vi "CSMKVMapDVR.vi"(8 "error in (no error)":errorcluster) -> (0 "error out":errorcluster, 3 "KVMapDVR":refnum<data-value>)   [LabVIEW 2017, in "Communicable State Machine.lvlib"]
uses:
  Communicable State Machine.lvlib
  ChangeFlag/ChangeFlag-Write.vi
  Utility/Random Change Flag.vi
  ChangeFlag/ChangeFlagDB.vi
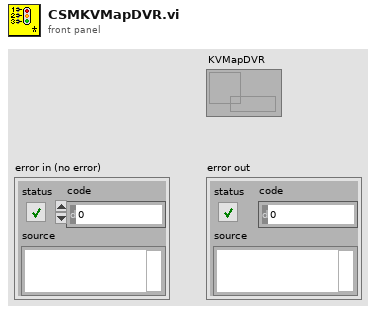
[diagram p1: front panel]
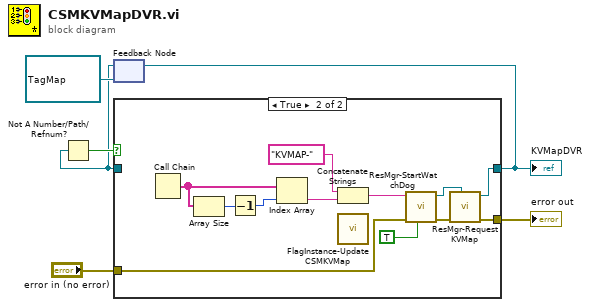
[diagram p0: block diagram]
diagram:
  n1 = feedback #1(refnum<data-value> refnum ("KVMapDVR")) -> (w3:refnum<data-value>)
  n2 = Not A Number/Path/Refnum?(number/path/refnum=w3) -> (NaN/Path/Refnum?=w4:bool)
  n3 = case shown="True" w4 {
    tunnel: w3 -> [w8 _]
    tunnel: [w8 w18] -> w6
    tunnel: [w7 w10] -> w2
    tunnel: "error in (no error)" -> [w7 w9]
    frame False {
    }
    frame True {
      n4 = Call Chain() -> (call chain=w13:string[])
      n5 = Array Size(array=w13) -> (size(s)=w12:i32)
      n6 = Decrement(x=w12) -> (x-1=w11:i32)
      n7 = Index Array(array=w13, index=w11) -> (element=w14:string)
      n8 = Concatenate Strings("KVMAP-" ("ModuleName"), w14) -> (w15:string)
      n9 = call "FlagInstance-Update CSMKVMap.vi"() -> ()  [unwired: 10 in, 2 out]
      n10 = call "ResMgr-StartWatchDog.vi"("Force?"=TRUE, "error in (no error)"=w9, "ModuleName"=w15) -> ("error out"=w19:errorcluster, "WatchDogQ"=w20:refnum<queue>)  [unwired: 7 in]
      n11 = call "ResMgr-Request KVMap.vi"("WatchDogQ"=w20, "Error In"=w19) -> ("error out"=w10:errorcluster, "KVMapDVR"=w18:refnum<data-value>)  [unwired: 8 in]
    }
  }
  "KVMapDVR" <- w6
  "error out" <- w2
  n12 = feedback-in #1(w6) -> ()
